vi "set_sample_number.vi"(8 "ERROR IN":errorcluster, 11 "EXP SETTINGS":refnum<notifier>) -> (0 "error out":errorcluster, 3 "EXP SETTINGS UPDATED":refnum<notifier>)   [LabVIEW 2013]
uses:
  type_defs/experiment_settings.ctl
  type_defs/experiment_states.ctl
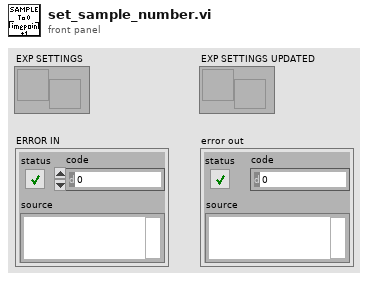
[diagram p1: front panel]
types:
  T1 = typedef "experiment_settings.ctl" = cluster{"fcs file byte offset":i64, "LED Device Handle Out":u32, "START TIME":timestamp, "CURRENT VALVE":u32, "SAMPLE #":i32, "FCS FILE PATH":path, "TIME POINT":i32, "STATE":T2, "TIME TILL SAMPLE":dbl, "DILUTION  TABLE":dbl[][]}
  T2 = typedef "experiment_states.ctl" = enum16{"OUTGROWTH", "INDUCTION", "EXPERIMENT"}
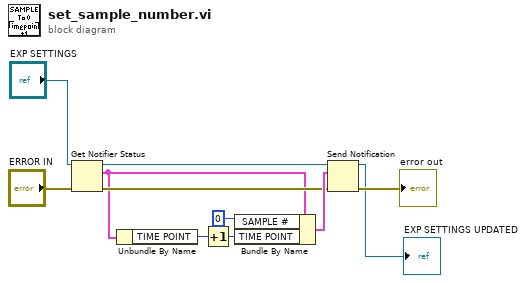
[diagram p0: block diagram]
diagram:
  n1 = Get Notifier Status(notifier="EXP SETTINGS", error in (no error)="ERROR IN") -> (notifier out=w6:refnum<notifier>, current notification=w3:T1, error out=w7:errorcluster)  [unwired: 2 out]
  n2 = Unbundle By Name(w3) -> ("TIME POINT"=w2:i32)
  n3 = Increment(x=w2) -> (x+1=w1:i32)
  n4 = Bundle By Name(cluster=w3, "SAMPLE #"=0, "TIME POINT"=w1) -> (w8:T1)
  n5 = Send Notification(notification=w8, notifier=w6, error in (no error)=w7) -> (notifier out=→"EXP SETTINGS UPDATED":refnum<notifier>, error out=→"error out":errorcluster)
